vi "PID version2.vi"(11 "Field Desired (T)":dbl) -> (3 "Tesla":dbl(knob) scale=0.0..1.25)   [LabVIEW 2009, in "Varian Magnet.lvclass"]
uses:
  Varian Magnet.lvclass
  <vilib>/DAQmx/create/channels.llb/DAQmx Create Channel (AO-Voltage-Basic).vi
  <vilib>/DAQmx/create/channels.llb/DAQmx Create Channel (AI-Voltage-Basic).vi
  <vilib>/DAQmx/write.llb/DAQmx Write (Analog DBL 1Chan 1Samp).vi
  <vilib>/Analysis/NI_AALBase.lvlib
panel:
  in  "stop":bool
  out "Actual Amps":dbl
  out "Waveform Chart 3":dynamicdata(graph)
  out "Waveform Chart 2":dbl(graph)
  in  "KD":dbl
  in  "KI":dbl
  in  "KP":dbl
  out "Amps Desired":dbl
  out "Waveform Chart":dbl(graph)
  out "Amps":dbl(knob) scale=0.0..1.5
  out "Raw voltage":dbl format="%0.4f"
  in  "data":dbl min=-9.0 max=9.0 format="%0.2f"
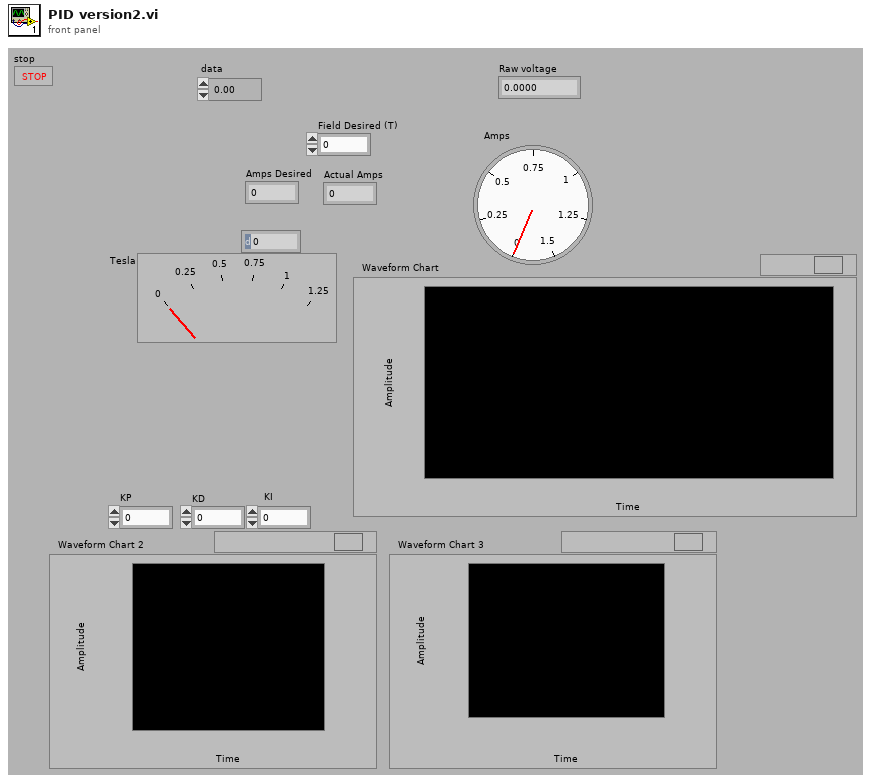
[diagram p1: front panel]
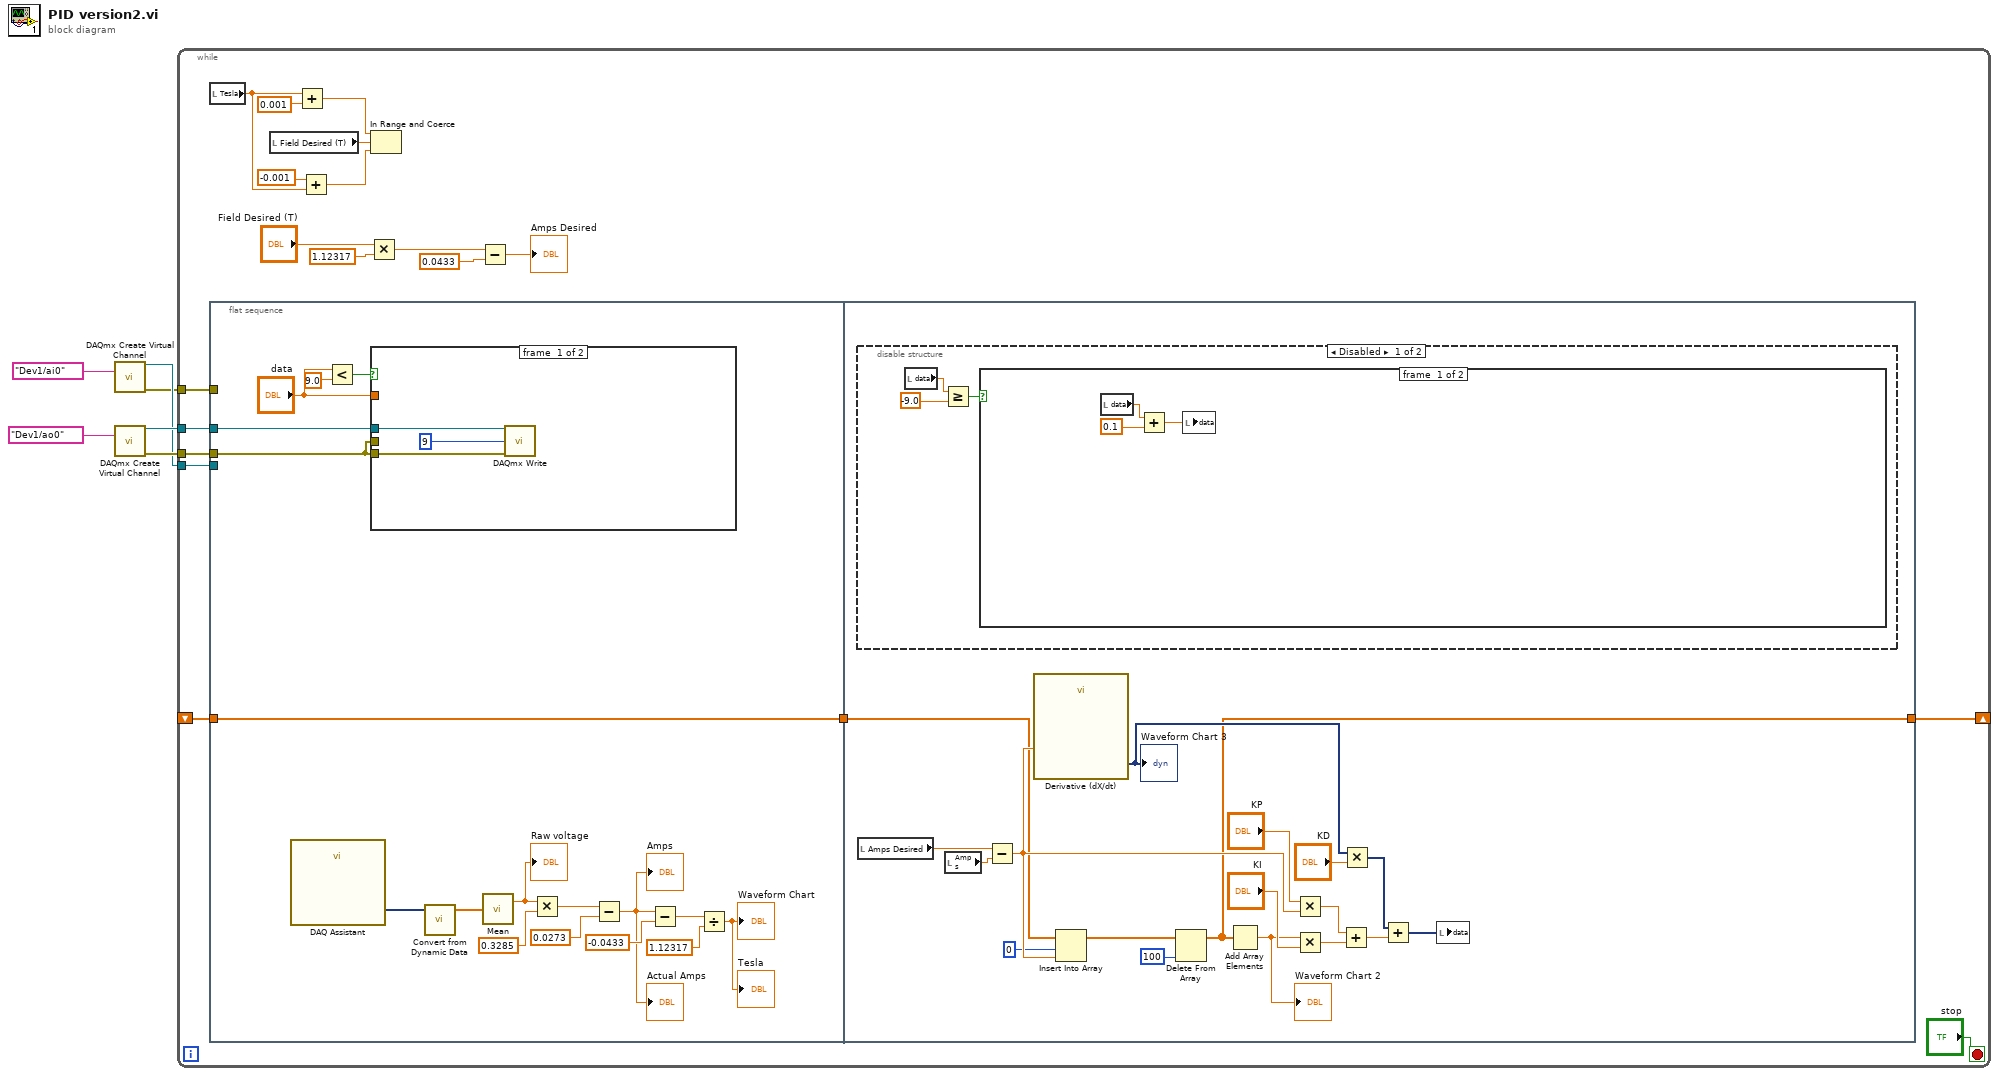
[diagram p0: block diagram]
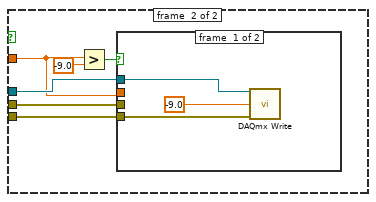
[diagram p2: hidden frame]
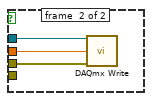
[diagram p3: hidden frame]
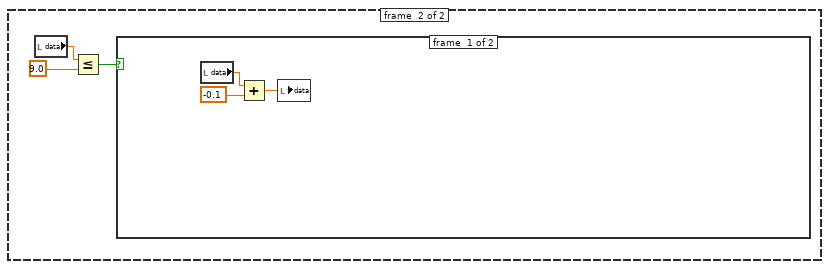
[diagram p4: hidden frame]
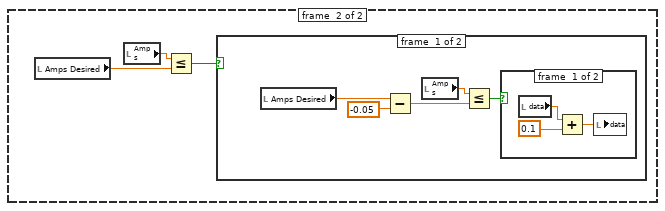
[diagram p5: hidden frame]
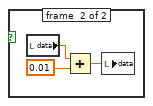
[diagram p6: hidden frame]
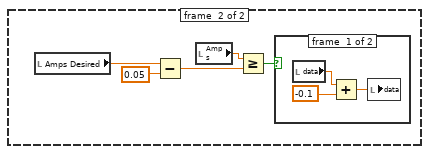
[diagram p7: hidden frame]
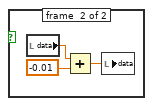
[diagram p8: hidden frame]
diagram:
  n1 = call-poly <vilib>:"DAQmx Create Virtual Channel.vi"("physical channels"=tag "Dev1/ai0") -> ("task out"=w3:refnum<k21>, "error out"=w2:errorcluster)  [unwired: 13 in]
  n2 = call-poly <vilib>:"DAQmx Create Virtual Channel.vi"("physical channels"=tag "Dev1/ao0") -> ("task out"=w5:refnum<k21>, "error out"=w4:errorcluster)  [unwired: 13 in]
  n3 = while {
    tunnel: w5 -> [w25]
    tunnel: w4 -> [w24]
    tunnel: w3 -> [w23]
    tunnel: w2 -> [w22]
    shift-right: [w16] -> _
    shift-left: _ -> [w15]
    stop <- "stop" stop-if-true
    n4 = local read "Tesla"() -> (w9:dbl)
    n5 = flat-sequence {
      tunnel: w25 -> [w42]
      tunnel: w24 -> [w32]
      tunnel: w23 -> [_]
      tunnel: w22 -> [_]
      tunnel: w15 -> [w26]
      tunnel: [w26] -> w14
      tunnel: [w60] -> w16
      tunnel: w14 -> [w59]
      frame #0 {
        n6 = call "DAQ Assistant"() -> ("data"=w41:dynamicdata)  [unwired: 17 in, 2 out]
        n7 = Less?(x="data", y=9.0) -> (x < y?=w29:bool)
        n8 = case shown="True" w29 {
          tunnel: w42 -> [w45 w51]
          tunnel: w32 -> [_ w50]
          tunnel: "data" -> [_ w46]
          tunnel: w32 -> [w44 w47]
          frame #0 {
            n9 = call-poly <vilib>:"DAQmx Write.vi"("task/channels in"=w45, "data"=9, "error in"=w44) -> ()  [unwired: 10 in, 3 out]
          }
          frame #1 {
            n10 = Greater?(x=w46, y=-9.0) -> (0:w49:bool)
            n11 = case shown="True" w49 {
              tunnel: w51 -> [w53 w57]
              tunnel: w50 -> [_ w56]
              tunnel: w46 -> [_ w55]
              tunnel: w47 -> [w54 _]
              frame #0 {
                n12 = call-poly <vilib>:"DAQmx Write.vi"("task/channels in"=w53, "data"=-9.0, "error in"=w54) -> ()  [unwired: 10 in, 3 out]
              }
              frame #1 {
                n13 = call-poly <vilib>:"DAQmx Write.vi"("task/channels in"=w57, "data"=w55, "error in"=w56) -> ()  [unwired: 10 in, 3 out]
              }
            }
          }
        }
        n14 = call "Convert from Dynamic Data"("Dynamic Data Type"=w41) -> ("Array"=w40:dbl[])  [unwired: 3 in]
        n15 = call <vilib>:"Mean.vi"("X"=w40) -> ("mean"=w39:dbl)  [unwired: 1 out]
        "Raw voltage" <- w39
        n16 = Multiply(x=w39, y=0.3285) -> (x*y=w37:dbl)
        n17 = Subtract(x=w37, y=0.0273) -> (x-y=w27:dbl)
        "Amps" <- w27
        "Actual Amps" <- w27
        n18 = Subtract(x=w27, y=-0.0433) -> (x-y=w33:dbl)
        n19 = Divide(x=w33, y=1.12317) -> (x/y=→"Waveform Chart" →"Tesla":dbl)
      }
      frame #1 {
        n20 = disable-structure shown="Disabled" {
          frame #0 {
            n21 = local read "data"() -> (w77:dbl)
            n22 = Greater Or Equal?(x=w77, y=-9.0) -> (x >= y?=w76:bool)
            n23 = case shown="True" w76 {
              frame #0 {
                n24 = local read "data"() -> (w80:dbl)
                n25 = Add(x=w80, y=0.1) -> (x+y=w79:dbl)
                n26 = local write "data"(w79) -> ()
              }
              frame #1 {
                n27 = local read "data"() -> (w84:dbl)
                n28 = Less Or Equal?(x=w84, y=9.0) -> (x <= y?=w82:bool)
                n29 = case shown="False" w82 {
                  frame #0 {
                    n30 = local read "data"() -> (w86:dbl)
                    n31 = Add(x=w86, y=-0.1) -> (x+y=w85:dbl)
                    n32 = local write "data"(w85) -> ()
                  }
                  frame #1 {
                    n33 = local read "Amps Desired"() -> (w88:dbl)
                    n34 = local read "Amps"() -> (w89:dbl)
                    n35 = Less Or Equal?(x=w89, y=w88) -> (x <= y?=w90:bool)
                    n36 = case shown="False" w90 {
                      frame #0 {
                        n37 = local read "Amps Desired"() -> (w92:dbl)
                        n38 = Subtract(x=w92, y=-0.05) -> (x-y=w93:dbl)
                        n39 = local read "Amps"() -> (w95:dbl)
                        n40 = Less Or Equal?(x=w95, y=w93) -> (x <= y?=w94:bool)
                        n41 = case shown="False" w94 {
                          frame #0 {
                            n42 = local read "data"() -> (w97:dbl)
                            n43 = Add(x=w97, y=0.1) -> (x+y=w96:dbl)
                            n44 = local write "data"(w96) -> ()
                          }
                          frame #1 {
                            n45 = local read "data"() -> (w100:dbl)
                            n46 = Add(x=w100, y=0.01) -> (x+y=w99:dbl)
                            n47 = local write "data"(w99) -> ()
                          }
                        }
                      }
                      frame #1 {
                        n48 = local read "Amps Desired"() -> (w103:dbl)
                        n49 = Subtract(x=w103, y=0.05) -> (x-y=w104:dbl)
                        n50 = local read "Amps"() -> (w106:dbl)
                        n51 = Greater Or Equal?(x=w106, y=w104) -> (x >= y?=w105:bool)
                        n52 = case shown="True" w105 {
                          frame #0 {
                            n53 = local read "data"() -> (w108:dbl)
                            n54 = Add(x=w108, y=-0.1) -> (x+y=w107:dbl)
                            n55 = local write "data"(w107) -> ()
                          }
                          frame #1 {
                            n56 = local read "data"() -> (w111:dbl)
                            n57 = Add(x=w111, y=-0.01) -> (x+y=w110:dbl)
                            n58 = local write "data"(w110) -> ()
                          }
                        }
                      }
                    }
                  }
                }
              }
            }
          }
          frame #1 {
          }
        }
        n59 = local read "Amps Desired"() -> (w75:dbl)
        n60 = local read "Amps"() -> (w74:dbl)
        n61 = Subtract(x=w75, y=w74) -> (x-y=w64:dbl)
        n62 = call "Derivative (dX/dt)"("Signals"=w64) -> ("Result"=w65:dynamicdata)  [unwired: 1 in, 5 out]
        "Waveform Chart 3" <- w65
        n63 = Insert Into Array(array=w59, index=0, new element=w64) -> (w63:dbl[])
        n64 = Delete From Array(array=w63, index=100) -> (array with subset deleted=w60:dbl[])  [unwired: 1 in, 1 out]
        n65 = Add Array Elements(numeric array=w60) -> (sum=w58:dbl)
        "Waveform Chart 2" <- w58
        n66 = Multiply(x="KP", y=w64) -> (x*y=w70:dbl)
        n67 = Multiply(x=w58, y="KI") -> (x*y=w69:dbl)
        n68 = Add(x=w70, y=w69) -> (x+y=w68:dbl)
        n69 = Multiply(x=w65, y="KD") -> (x*y=w67:dynamicdata)
        n70 = Add(x=w67, y=w68) -> (x+y=w66:dynamicdata)
        n71 = local write "data"(w66) -> ()
      }
    }
    n72 = local read "Field Desired (T)"() -> (w13:dbl)
    n73 = Add(x=w9, y=0.001) -> (x+y=w11:dbl)
    n74 = Add(x=-0.001, y=w9) -> (x+y=w12:dbl)
    n75 = Multiply(x="Field Desired (T)", y=1.12317) -> (x*y=w21:dbl)
    n76 = In Range and Coerce(upper limit=w11, x=w13, lower limit=w12) -> ()  [unwired: 2 out]
    n77 = Subtract(x=w21, y=0.0433) -> (x-y=→"Amps Desired":dbl)
  }
